vi "Lab.08_BP.vi"() -> ()   [LabVIEW 2016]
panel:
  out "amplitude":dbl
  out "MIC":dynamicdata(graph)
  out "Pressure":dynamicdata(graph)
  in  "stop":bool
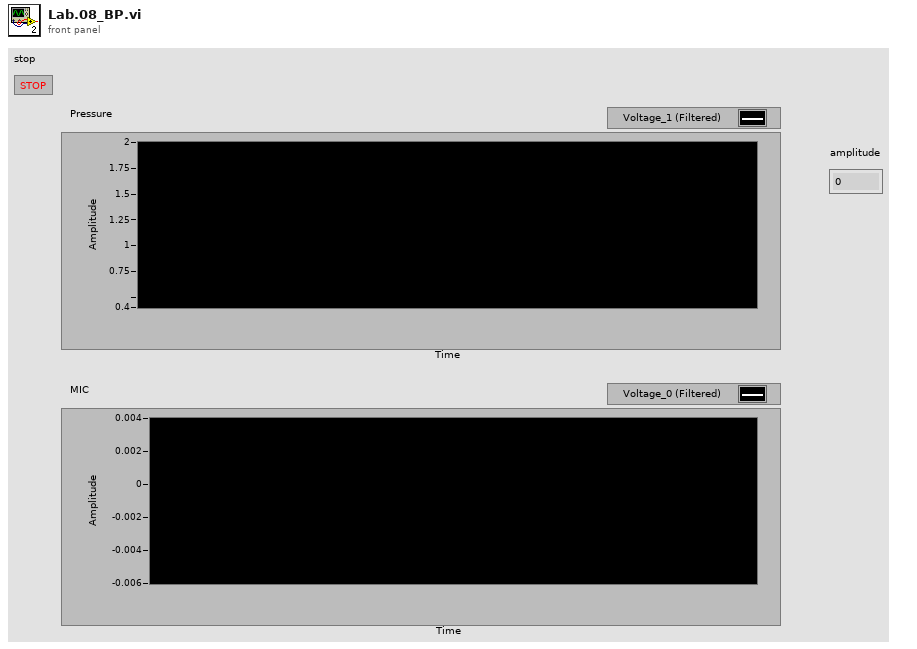
[diagram p1: front panel]
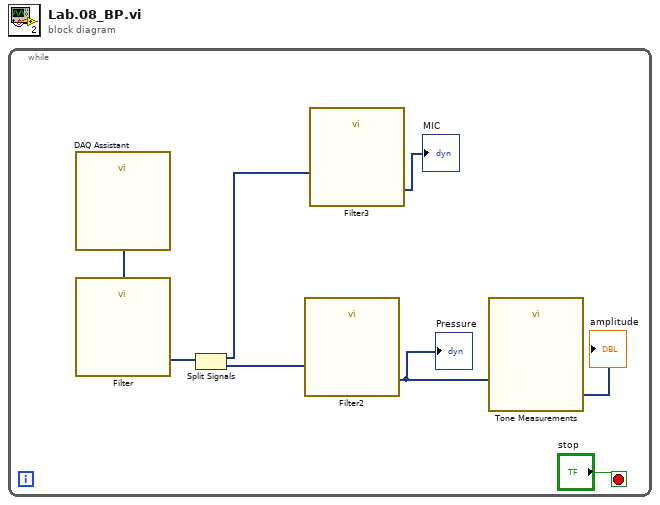
[diagram p0: block diagram]
diagram:
  n1 = while {
    stop <- "stop" stop-if-true
    n2 = call "DAQ Assistant"() -> ("data"=w7:dynamicdata)  [unwired: 16 in, 3 out]
    n3 = call "Filter"("Signal"=w7) -> ("Filtered Signal"=w6:dynamicdata)  [unwired: 9 in, 1 out]
    n4 = Split Signals(w6) -> (w3:dynamicdata, w4:dynamicdata)  [unwired: 2 in]
    n5 = call "Filter2"("Signal"=w4) -> ("Filtered Signal"=w2:dynamicdata)  [unwired: 9 in, 1 out]
    "Pressure" <- w2
    n6 = call "Filter3"("Signal"=w3) -> ("Filtered Signal"=→"MIC":dynamicdata)  [unwired: 9 in, 1 out]
    n7 = call "Tone Measurements"("Signals"=w2) -> ("Amplitude"=→"amplitude":dynamicdata)  [unwired: 9 in, 1 out]
  }
